vi "Filtered Gaussian WN Ident.vi"() -> ()   [LabVIEW 2015]
uses:
  <vilib>/Analysis/3filter.llb/Filter Passband Type.ctl
  <vilib>/Platform/TimedLoop/XDataNode/timing_clust.ctl
  <vilib>/Platform/TimedLoop/XDataNode/nitl_modes.ctl
  <vilib>/Platform/TimedLoop/XDataNode/wakeup.ctl
  <vilib>/Analysis/2dsp.llb/Power Spectrum (DBL).vi
  <vilib>/Analysis/2dsp.llb/1D Auto Correlation (DBL).vi
  <vilib>/FPGAPlugInAG/myRIO-1900/niLvFpga_Open_myRIO-1900.vi
  <vilib>/rvi/interface/common/dynamic/niFpgaDynamicAddResources.vi
  <vilib>/Utility/file.llb/Write Delimited Spreadsheet (DBL).vi
  <vilib>/Utility/error.llb/Error Cluster From Error Code.vi
  <vilib>/rvi/errors/niLvFpgaAdjustHostInterfaceError.vi
  <vilib>/FPGAPlugInAG/Dynamic/niLvFpga_Close_Dynamic.vi
  <vilib>/rvi/interface/nirviOpenFPGA/nirviOpenFPGA.xnode
  FPGA Bitfiles/ViconProj_FPGATarget_CurrentControlle_KJVtLDFLiQk.lvbitx
  Misc/Current Controller.vi
  <vilib>/Platform/TimedLoop/XDataNode/XDataNode.xnode
  <vilib>/rvi/interface/nirviReadWriteControl/nirviReadWriteControl.xnode
  <vilib>/rvi/interface/nirviCloseFPGA/nirviCloseFPGA.xnode
  <vilib>/rvi/interface/Simulation/niFpgaSimulationCallBeginRW.vi
  <vilib>/Platform/TimedLoop/XDataNode/XDNodeRunTimeDep.lvlib
  <vilib>/Analysis/NI_AALBase.lvlib
  <vilib>/Analysis/NI_AALPro.lvlib
  <vilib>/ptbypt/NI_PtbyPt.lvlib
  NiFpgaLv.dll
panel:
  out "Pose":dbl[][](array[numeric])
  in  "Tab Control 2":enum32{"Page 1"}(tab)
  in  "Stop":bool
  in  "ACF normalization":enum32{"none", "unbiased", "biased"}(ring)=enum."unbiased"
  in  "std dev":dbl(knob)=16.254291221099862 scale=0.0..20.0
  in  "filter type":T1=enum."Bandpass"
  in  "window":T2(ring)=enum."Exact Blackman"
  in  "taps":i32(slide)=18 scale=0.0..25.0
  in  "low cutoff freq: fl":dbl(knob)=100.0 scale=5.0..6.0
  in  "high cutoff freq: fh":dbl(knob)=0.45 scale=0.0..12.0
  in  "Tab Control":enum32{"Monitor", "Monitor 2"}(tab)
  out "GWN Wave":dbl[](graph)
  out "FPGA Status":bool
  out "Power Spectrum":dbl[](graph)
  out "error":i32
  out "GWN Filtered":dbl[](graph)
  out "In Range?":bool[](array[boolean])
  out "Crest Factor":dbl[](graph)
  out "yaw":dbl
  out "pitch":dbl
  out "roll":dbl
  out "y":dbl
  out "z":dbl
  out "x":dbl
  out "PoseVect":dbl[][](graph)
  out "FPGA Loop error":errorcluster
  out "FPGA TImed Loop error":errorcluster
  out "UWGN Error":errorcluster
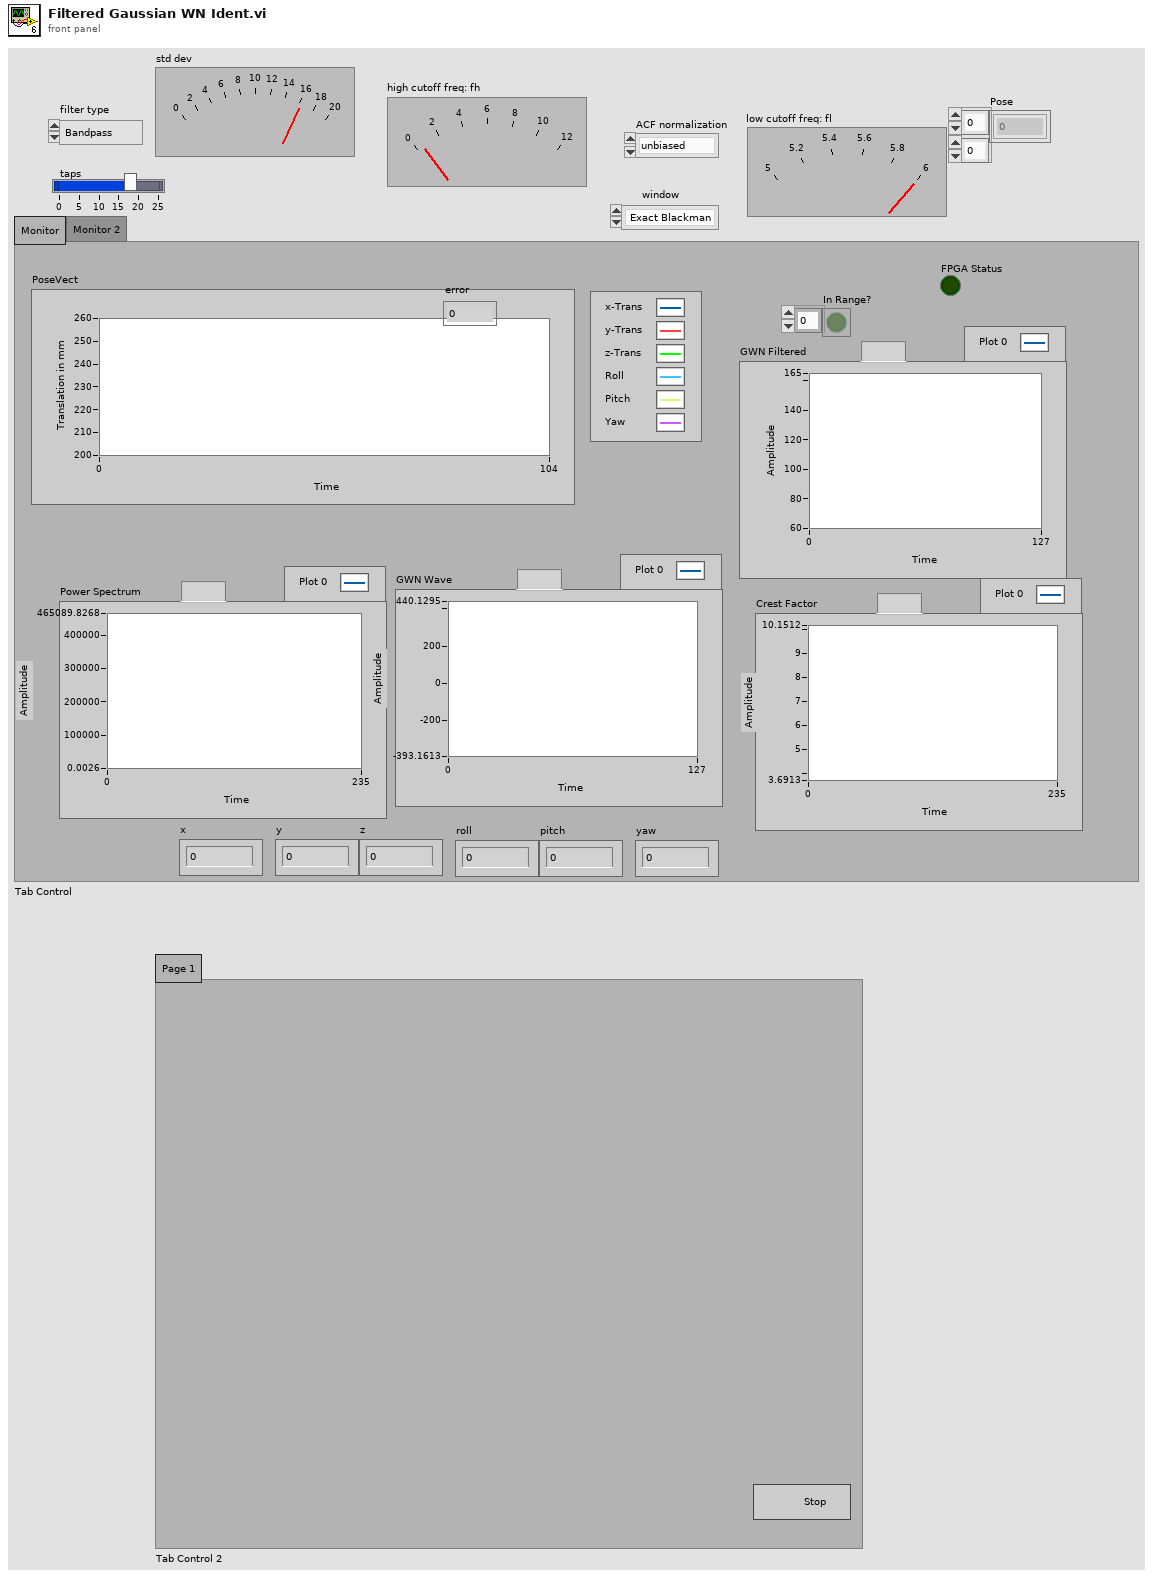
[diagram p1: front panel]
types:
  T1 = typedef "NI_AALBase.lvlib/Filter Passband Type.ctl" = enum32{"Lowpass", "Highpass", "Bandpass", "Bandstop"}
  T2 = enum32{"None", "Hanning", "Hamming", "Triangular", "Blackman", "Exact Blackman", "Blackman-Harris", "Kaiser-Bessel", "Flat Top"}
  T3 = typedef "XDNodeRunTimeDep.lvlib/timing_clust.ctl" = cluster{"Expected End [f-1]":u64, "Actual End [f-1]":u64, "Finished Late? [f-1]":bool, "Expected End [i-1]":u64, "Actual End [i-1]":u64, "Finished Late? [i-1]":bool, "Expected Start [i]":u64, "Actual Start [i]":u64, "Expected Start [f]":u64, "Actual Start [f]":u64, "Source Name":string, "Structure Name":string, "Period":i64, "Deadline":i64, "Offset":i64, "Start":i64, "Priority":i32, "Timeout":i32, "Mode":T4, "Wakeup Reason":T5, "Error":errorcluster, "Source Type":string, "Secondary Source Type":string, "Global End Time":u64, "Global Start Time":u64, "Frame Duration":u64, "Iteration Duration":u64, "Assigned CPU":i32, "I/O Scan Engine Mode":u32}
  T4 = typedef "XDNodeRunTimeDep.lvlib/nitl_modes.ctl" = enum32{"No Change", "Process missed periods, maintain original phase", "Discard missed periods, maintain original phase", "Process missed periods, ignore original phase", "Discard missed periods, ignore original phase"}
  T5 = typedef "XDNodeRunTimeDep.lvlib/wakeup.ctl" = enum32{"Normal", "Aborted", "Asynchronous wakeup", "Timing source error", "Timed loop error", "Timeout"}
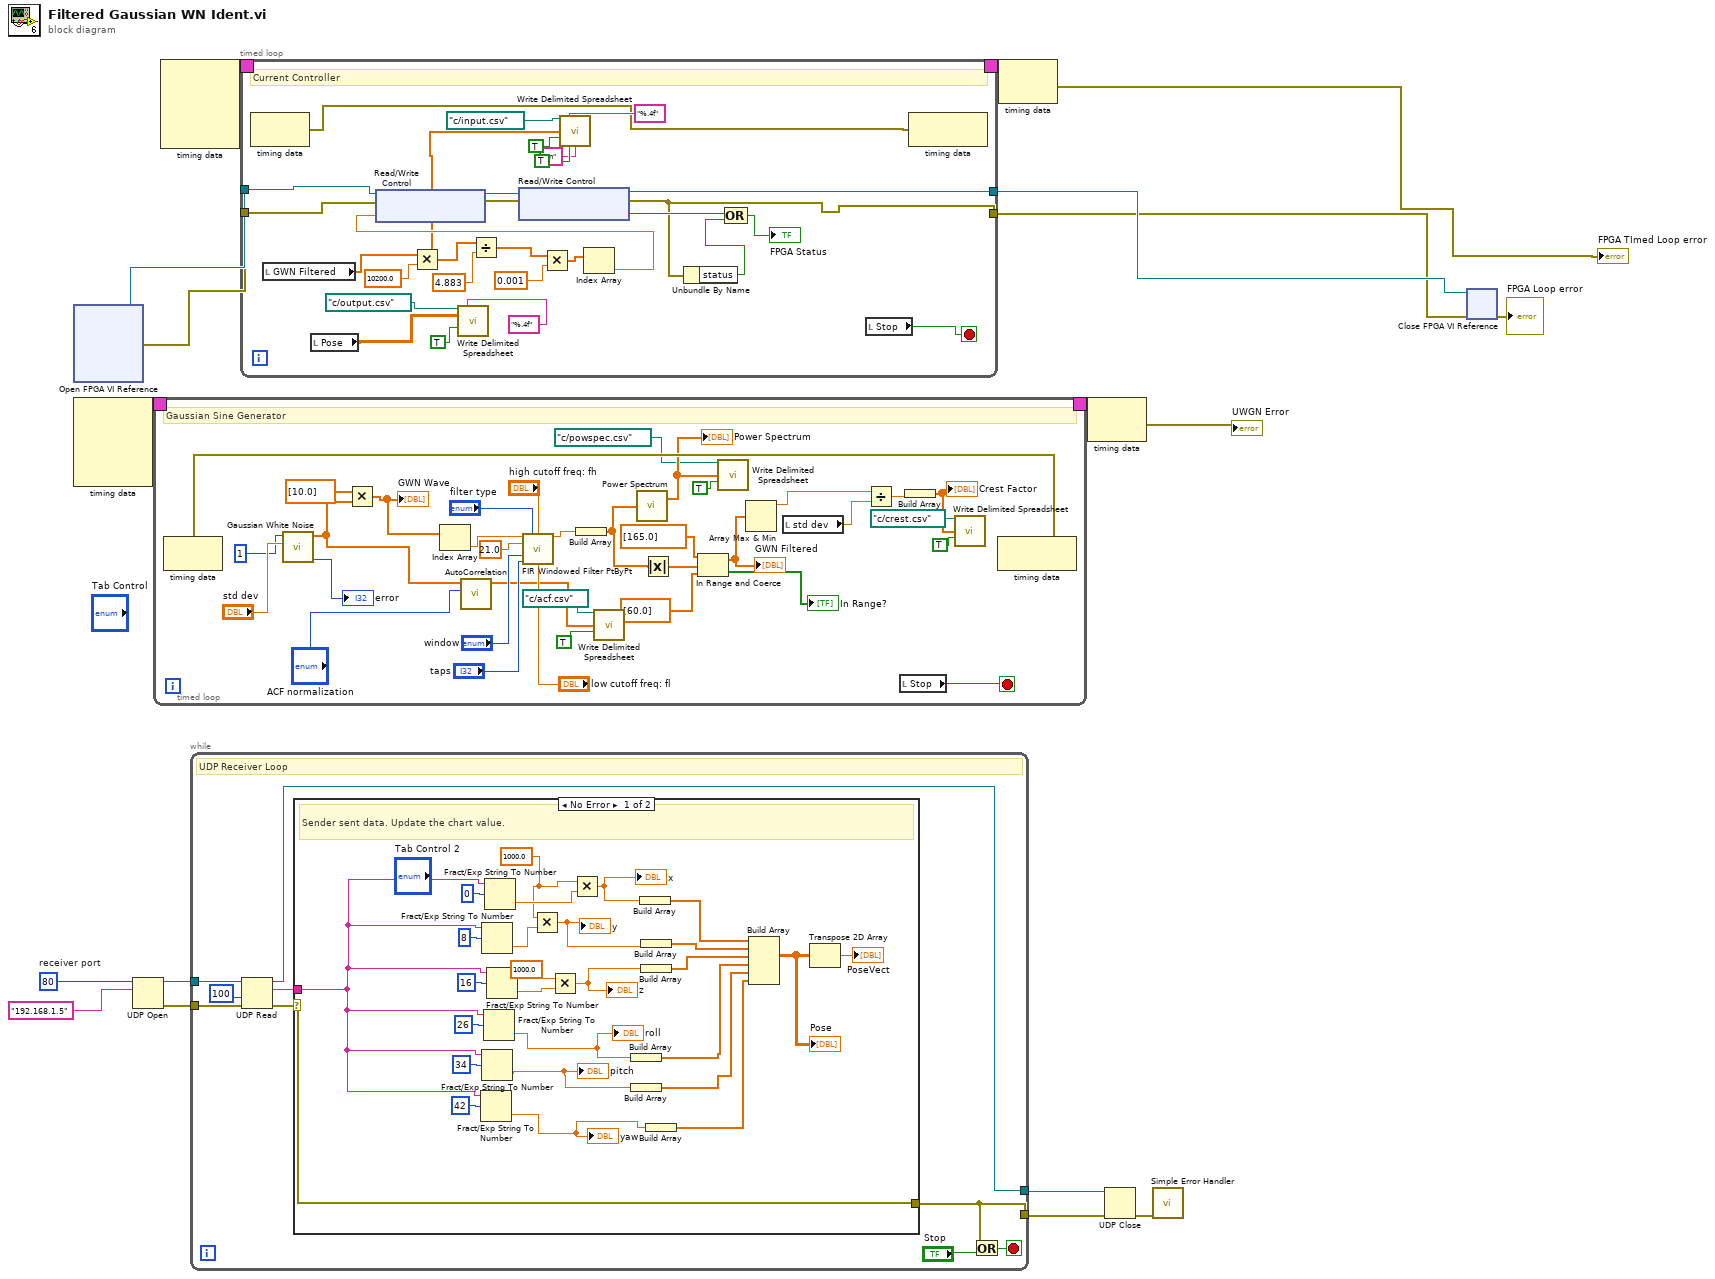
[diagram p0: block diagram]
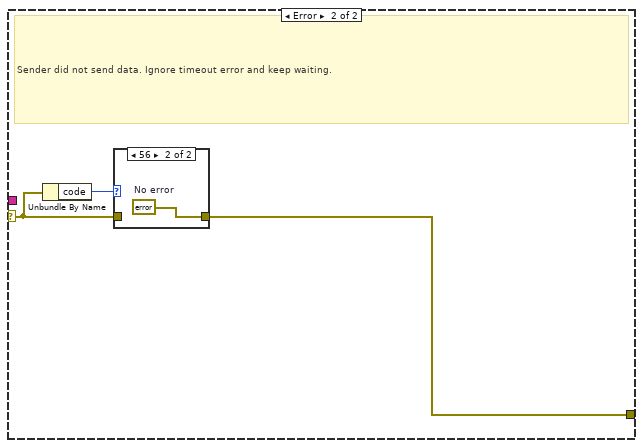
[diagram p2: hidden frame]
diagram:
  w2 = u16 80  # receiver port
  n1 = xnode "Open FPGA VI Reference"() -> ("FPGA VI Reference Out"=w18:refnum<k20>, "error out"=w17:errorcluster)  [unwired: 2 in]
  n2 = node-c288() -> (w14:T3)  [unwired: 4 in]
  n3 = UDP Open(10:"192.168.1.5" ("service name"), 11:w2) -> (port=w3:refnum<k16>, 0:w4:errorcluster)  [unwired: 3 in, 1 out]
  n4 = timed-loop {
    timing: w14 -> [_]
    timing-out: [_] -> w13
    stop <- w24 stop-if-true
    # "Gaussian Sine Generator"
    n5 = node-c288() -> (w53:errorcluster)  [unwired: 1 in]
    n6 = call <vilib>:"Gaussian White Noise.vi"("standard deviation"="std dev", "samples"=1) -> ("error"=→"error":i32, "Gaussian noise pattern"=w21:dbl[])  [unwired: 8 in]
    n7 = Multiply(x=dbl[] [10.0], y=w21) -> (x*y=w19:dbl[])
    "GWN Wave" <- w19
    n8 = Index Array(array=w19) -> (element=w46:dbl)  [unwired: 1 in]
    n9 = call-poly <vilib>:"AutoCorrelation.vi"("normalization"="ACF normalization", "X"=w21) -> ("Rxx"=w29:dbl[])  [unwired: 8 in, 1 out]
    n10 = call <vilib>:"FIR Windowed Filter PtByPt.vi"("x"=w46, "filter type"="filter type", "high cutoff freq: fh"="high cutoff freq: fh", "sampling freq: fs"=21.0, "window"="window", "taps"="taps", "low cutoff freq: fl"="low cutoff freq: fl") -> ("Filtered x"=w41:dbl)  [unwired: 7 in, 1 out]
    n11 = Build Array(w41) -> (w23:dbl[])
    n12 = call-poly <vilib>:"Write Delimited Spreadsheet.vi"("file path (dialog if empty)"=path "c:/acf.csv", "1D data"=w29, "append to file? (F)"=TRUE) -> ()  [unwired: 11 in, 2 out]
    n13 = call-poly <vilib>:"Power Spectrum.vi"("X"=w23) -> ("Power Spectrum"=w27:dbl[])  [unwired: 1 out]
    "Power Spectrum" <- w27
    n14 = Absolute Value(x=w23) -> (abs(x)=w22:dbl[])
    n15 = In Range and Coerce(upper limit=dbl[] [165.0], x=w22, lower limit=dbl[] [60.0]) -> (coerced(x)=w37:dbl[], In Range?=→"In Range?":bool[])
    "GWN Filtered" <- w37
    n16 = call-poly <vilib>:"Write Delimited Spreadsheet.vi"("file path (dialog if empty)"=path "c:/powspec.csv", "1D data"=w27, "append to file? (F)"=TRUE) -> ()  [unwired: 11 in, 2 out]
    n17 = Array Max & Min(array=w37) -> (max value=w36:dbl)  [unwired: 3 out]
    n18 = local read "std dev"() -> (w35:dbl)
    n19 = Divide(x=w36, y=w35) -> (x/y=w34:dbl)
    n20 = local read "Stop"() -> (w24:bool)
    n21 = Build Array(w34) -> (w33:dbl[])
    "Crest Factor" <- w33
    n22 = call-poly <vilib>:"Write Delimited Spreadsheet.vi"("file path (dialog if empty)"=path "c:/crest.csv", "1D data"=w33, "append to file? (F)"=TRUE) -> ()  [unwired: 11 in, 2 out]
    n23 = node-c288(w53) -> ()  [unwired: 1 out]
  }
  n24 = node-c288() -> (w12:T3)  [unwired: 4 in]
  n25 = while {
    tunnel: w3 -> [w67]
    tunnel: [w59] -> w7
    tunnel: w4 -> [w64]
    tunnel: [w60] -> w5
    stop <- w65 stop-if-true
    # "UDP Receiver Loop"
    n26 = UDP Read(connection ID=w67, timeout ms (25000)=100, 8:w64) -> (data out=w62:string, error out=w61:errorcluster, 3:w59:refnum<k16>)  [unwired: 3 out]
    n27 = case shown="No Error" w61 {
      selector: w61 -> [w94 w96]
      tunnel: w62 -> [w77 _]
      tunnel: [w94 w95] -> w60
      frame No Error {
        w76 = 1000.0 ("y")
        # "Sender sent data. Update the chart value."
        n28 = Fract/Exp String To Number(string=w77, offset=42) -> (number=w68:dbl)  [unwired: 2 in, 1 out]
        "yaw" <- w68
        n29 = Fract/Exp String To Number(string=w77, offset=8) -> (number=w80:dbl)  [unwired: 2 in, 1 out]
        n30 = Fract/Exp String To Number(string=w77, offset=34) -> (number=w69:dbl)  [unwired: 2 in, 1 out]
        "pitch" <- w69
        n31 = Fract/Exp String To Number(string=w77, offset=26) -> (number=w70:dbl)  [unwired: 2 in, 1 out]
        "roll" <- w70
        n32 = Fract/Exp String To Number(string=w77, offset=0) -> (number=w83:dbl)  [unwired: 2 in, 1 out]
        n33 = Fract/Exp String To Number(string=w77, offset=16) -> (number=w82:dbl)  [unwired: 2 in, 1 out]
        n34 = Multiply(x=w76, y=w80) -> (x*y=w79:dbl)
        "y" <- w79
        n35 = Multiply(x=1000.0, y=w82) -> (x*y=w78:dbl)
        "z" <- w78
        n36 = Multiply(x=w76, y=w83) -> (x*y=w84:dbl)
        "x" <- w84
        n37 = Build Array(w70) -> (w73:dbl[])
        n38 = Build Array(w69) -> (w72:dbl[])
        n39 = Build Array(w84) -> (w86:dbl[])
        n40 = Build Array(w79) -> (w85:dbl[])
        n41 = Build Array(w78) -> (w90:dbl[])
        n42 = Build Array(w68) -> (w71:dbl[])
        n43 = Build Array(w86, w85, w90, w73, w72, w71) -> (w75:dbl[][])
        "Pose" <- w75
        n44 = Transpose 2D Array(2D array=w75) -> (transposed array=→"PoseVect":dbl[][])
      }
      frame Error {
        # "Sender did not send data. Ignore timeout error and keep waiting."
        n45 = Unbundle By Name(w96) -> ("code"=w97:i32)
        n46 = case shown="56" w97 {
          tunnel: w96 -> [w98 _]
          tunnel: [w98 w99] -> w95
          frame Default {
          }
          frame 56 {
            w99 = errorcluster {"status"=FALSE, "code"=0, "source"=""}  # No error
          }
        }
      }
    }
    n47 = Or(x=w60, y="Stop") -> (x .or. y?=w65:bool)
  }
  n48 = timed-loop {
    tunnel: w18 -> [w127]
    tunnel: w17 -> [w126]
    tunnel: [w118] -> w16
    tunnel: [w115] -> w15
    timing: w12 -> [_]
    timing-out: [_] -> w11
    stop <- w101 stop-if-true
    # "Current Controller"
    n49 = node-c288() -> (w105:errorcluster)  [unwired: 1 in]
    n50 = local read "GWN Filtered"() -> (w102:dbl[])
    n51 = local read "Pose"() -> (w100:dbl[][])
    n52 = Multiply(x=w102, y=10200.0) -> (x*y=w122:dbl[])
    n53 = call-poly <vilib>:"Write Delimited Spreadsheet.vi"("file path (dialog if empty)"=path "c:/output.csv", "format (%.3f)"="%.4f", "2D data"=w100, "append to file? (F)"=TRUE) -> ()  [unwired: 10 in, 2 out]
    n54 = Divide(x=w122, y=4.883) -> (x/y=w124:dbl[])
    n55 = Multiply(x=w124, y=0.001) -> (x*y=w107:dbl[])
    n56 = call-poly <vilib>:"Write Delimited Spreadsheet.vi"("file path (dialog if empty)"=path "c:/input.csv", "format (%.3f)"="%.4f" ("format (%d)"), "1D data"=w102, "append to file? (F)"=TRUE, "transpose? (F)"=TRUE, "delimiter (\\t)"="\\n" ("delimiter (\\t)")) -> ()  [unwired: 8 in, 2 out]
    n57 = Index Array(array=w107) -> (element=w106:dbl)  [unwired: 1 in]
    n58 = xnode "Read/Write Control"("FPGA VI Reference In"=w127, "error in"=w126, "DAC Outlet Valve"=w106) -> ("FPGA VI Reference Out"=w120:refnum<k20>, "error out"=w119:errorcluster)
    n59 = xnode "Read/Write Control"("FPGA VI Reference In"=w120, "error in"=w119) -> ("FPGA VI Reference Out"=w118:refnum<k20>, "error out"=w115:errorcluster, "Outlet Overflow?"=w116:bool)
    n60 = Unbundle By Name(w115) -> ("status"=w117:bool)
    n61 = Compound Arithmetic op=OR(w116, w117) -> (→"FPGA Status":bool)
    n62 = local read "Stop"() -> (w101:bool)
    n63 = node-c288(w105) -> ()  [unwired: 1 out]
  }
  n64 = node-c288(w11) -> (→"FPGA TImed Loop error":errorcluster)
  n65 = node-c288(w13) -> (→"UWGN Error":errorcluster)
  n66 = UDP Close(connection ID=w7, 8:w5) -> (error out=w6:errorcluster)  [unwired: 1 out]
  n67 = call <vilib>:"Simple Error Handler.vi"("error in (no error)"=w6) -> ()  [unwired: 1 in, 8 out]
  n68 = xnode "Close FPGA VI Reference"("FPGA VI Reference In"=w16, "error in"=w15) -> ("error out"=→"FPGA Loop error":errorcluster)
